vi "Set and Measure ITEMP.vi"(4 "Header":string="HighVsec", 6 "Name":string, 7 "Position in":u32, 8 "error in (no error)":errorcluster, 9 "Measurement Wait Time":u32, 10 "Cree Comms in":refnum<class "Cree Communications.lvclass">, 11 "Calibration in":refnum<class "Calibration.lvclass">) -> (0 "error out":errorcluster, 2 "DSpic Measurement":dbl, 3 "Actual Measurement":dbl)   [LabVIEW 2015, in "Calibration.lvclass"]
uses:
  Calibration.lvclass
  Classes/Cree Communications/Class/Cree Communications.lvclass
  Classes/Instruments/Power Supply/Class/Power Supply.lvclass
  Test Class/Test Class.lvclass
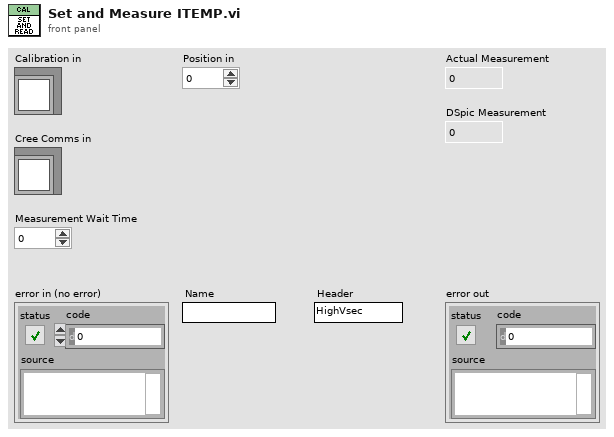
[diagram p1: front panel]
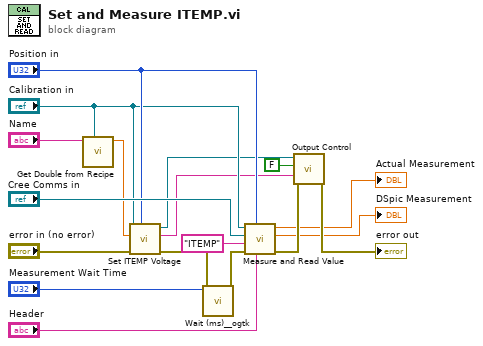
[diagram p0: block diagram]
diagram:
  n1 = call "Get Double from Recipe.vi"("Test Class in"="Calibration in", "Name"="Name") -> ("Value"=w4:dbl)  [unwired: 7 in, 2 out]
  n2 = call "Set ITEMP Voltage.vi"("Position in"="Position in", "Error in"="error in (no error)", "Voltage"=w4, "Calibration in"="Calibration in") -> ("Error out"=w7:errorcluster, "Channel"=w3:string, "Power Supply"=w2:refnum<class "Power Supply.lvclass">)  [unwired: 5 in]
  n3 = call <userlib>:"Wait (ms)__ogtk.vi"("error in (no error)"=w7, "milliseconds to wait"="Measurement Wait Time") -> ("error out"=w14:errorcluster)  [unwired: 8 in, 1 out]
  n4 = call "Measure and Read Value.vi"("Header"="Header", "Position"="Position in", "error in (no error)"=w14, "Calibration Type"="ITEMP", "Cree Communications"="Cree Comms in", "Calibration in"="Calibration in") -> ("error out"=w18:errorcluster, "DSpic Measurement"=→"DSpic Measurement":dbl, "Actual Measurement"=→"Actual Measurement":dbl)  [unwired: 3 in]
  n5 = call-dynamic "Output Control.vi"("Channel (\"1\")"=w3, "error in (no error)"=w18, "Enabled"=FALSE, "Acrobat Template in"=w2) -> ("error out"=→"error out":errorcluster)  [unwired: 6 in, 1 out]
